vi "AF Customer.vi"() -> ()   [LabVIEW 2020]
uses:
  Program Files (x86)/National Instruments/LabVIEW 2020/examples/Design Patterns/Actor Framework/Classes/Customer/Customer.lvclass
  C:/Program Files (x86)/National Instruments/LabVIEW 2020/vi.lib/ActorFramework/Actor/Actor.lvclass
  Program Files (x86)/National Instruments/LabVIEW 2020/examples/Design Patterns/Actor Framework/Classes/Beverages/Beverage/Beverage.lvclass
  Program Files (x86)/National Instruments/LabVIEW 2020/examples/Design Patterns/Actor Framework/Classes/Person Messages/Show or Hide Front Panel Msg/Show or Hide Front Panel Msg.lvclass/Show or Hide Front Panel Msg.ctl
  <vilib>/ActorFramework/Message Enqueuer/Message Enqueuer.lvclass/Message Enqueuer.ctl
  Program Files (x86)/National Instruments/LabVIEW 2020/examples/Design Patterns/Actor Framework/Classes/Customer Messages/Pick up Item Msg/Pick up Item Msg.lvclass/Pick up Item Msg.ctl
  <vilib>/ActorFramework/Message Enqueuer/Enqueue.vi
  Program Files (x86)/National Instruments/LabVIEW 2020/examples/Design Patterns/Actor Framework/Classes/Person Messages/Show or Hide Front Panel Msg/Show or Hide Front Panel Msg.lvclass
  C:/Program Files (x86)/National Instruments/LabVIEW 2020/vi.lib/ActorFramework/Message/Message.lvclass
  Program Files (x86)/National Instruments/LabVIEW 2020/examples/Design Patterns/Actor Framework/Classes/Customer Messages/Pick up Item Msg/Pick up Item Msg.lvclass
  <vilib>/ActorFramework/Stop Msg/Stop Msg.lvclass
  <vilib>/ActorFramework/Message Priority Queue/Priority Enqueue.vi
  <vilib>/ActorFramework/Actor/Actor.lvclass
panel:
  out "error out":errorcluster
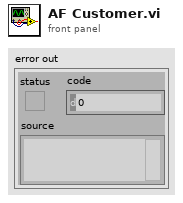
[diagram p1: front panel]
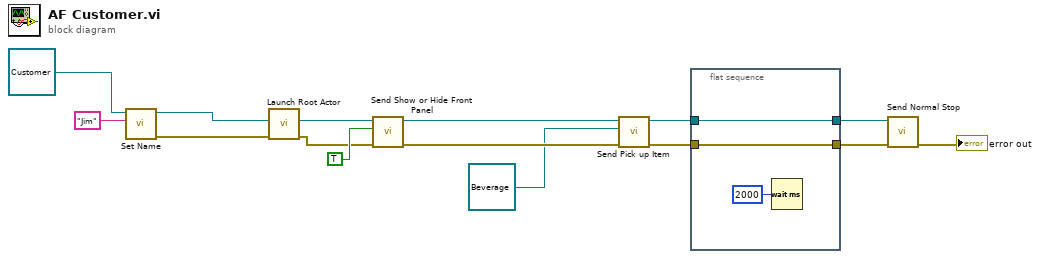
[diagram p0: block diagram]
diagram:
  n1 = call-dynamic "Set Name.vi"("Name"="Jim", "Person in"=refnum<class "Customer.lvclass"> refnum ("Customer.lvlib:Customer.lvclass")) -> ("error out"=w7:errorcluster, "Person out"=w5:refnum<class "Customer.lvclass">)  [unwired: 8 in]
  n2 = call <vilib>:"Launch Root Actor.vi"("error in (no error)"=w7, "Actor"=w5) -> ("error out"=w9:errorcluster, "Actor's Enqueuer"=w14:refnum<class "Message Enqueuer.lvclass">)  [unwired: 8 in]
  n3 = call "Send Show or Hide Front Panel.vi"("error in (no error)"=w9, "Show Front Panel?"=TRUE, "Message Enqueuer"=w14) -> ("error out"=w8:errorcluster, "Message Enqueuer out"=w4:refnum<class "Message Enqueuer.lvclass">)  [unwired: 7 in]
  n4 = call "Send Pick up Item.vi"("error in (no error)"=w8, "Beverage.lvclass"=refnum<class "Beverage.lvclass"> refnum, "Message Enqueuer"=w4) -> ("error out"=w2:errorcluster, "Message Enqueuer out"=w3:refnum<class "Message Enqueuer.lvclass">)  [unwired: 7 in]
  n5 = flat-sequence {
    tunnel: [w17] -> w15
    tunnel: w3 -> [w17]
    tunnel: [w16] -> w6
    tunnel: w2 -> [w16]
    frame #0 {
      n6 = Wait (ms)(milliseconds to wait=u32 2000) -> ()  [unwired: 1 out]
    }
  }
  n7 = call <vilib>:"Send Normal Stop.vi"("error in (no error)"=w6, "Message Enqueuer"=w15) -> ("error out"=→"error out":errorcluster)  [unwired: 9 in]
